vi "生成文本文件.vi"() -> ()   [LabVIEW 2013]
uses:
  <vilib>/Utility/file.llb/Write To Spreadsheet File (string).vi
panel:
  in  "字符串":string="1"
  in  "产品ID":string="201209190001"
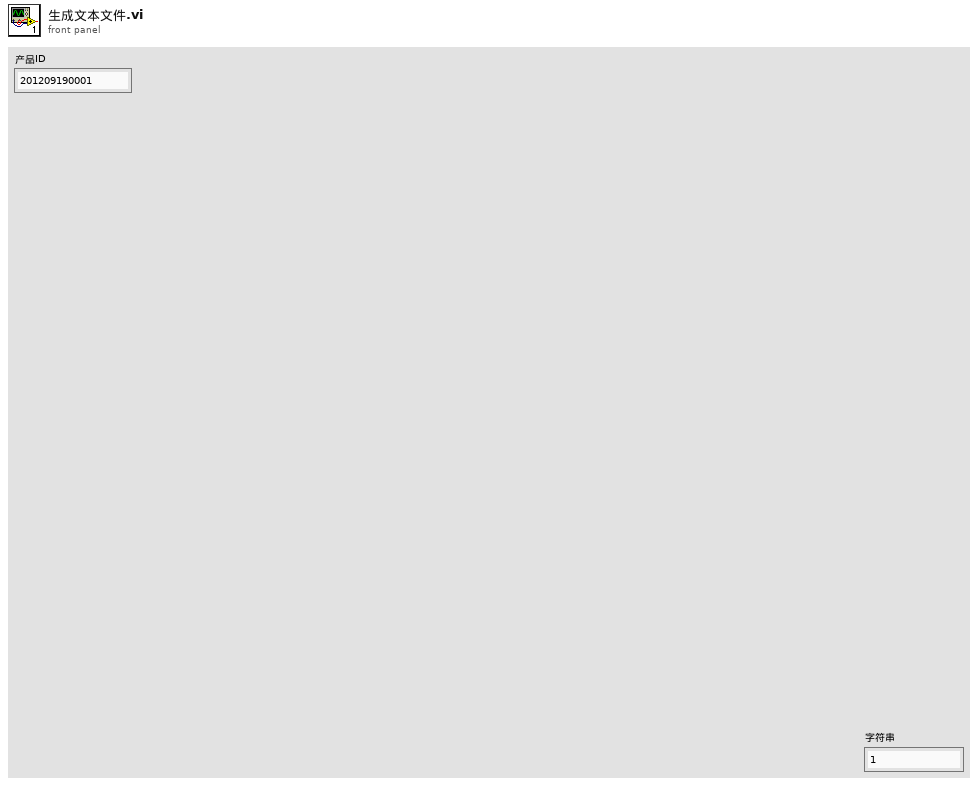
[diagram p1: front panel]
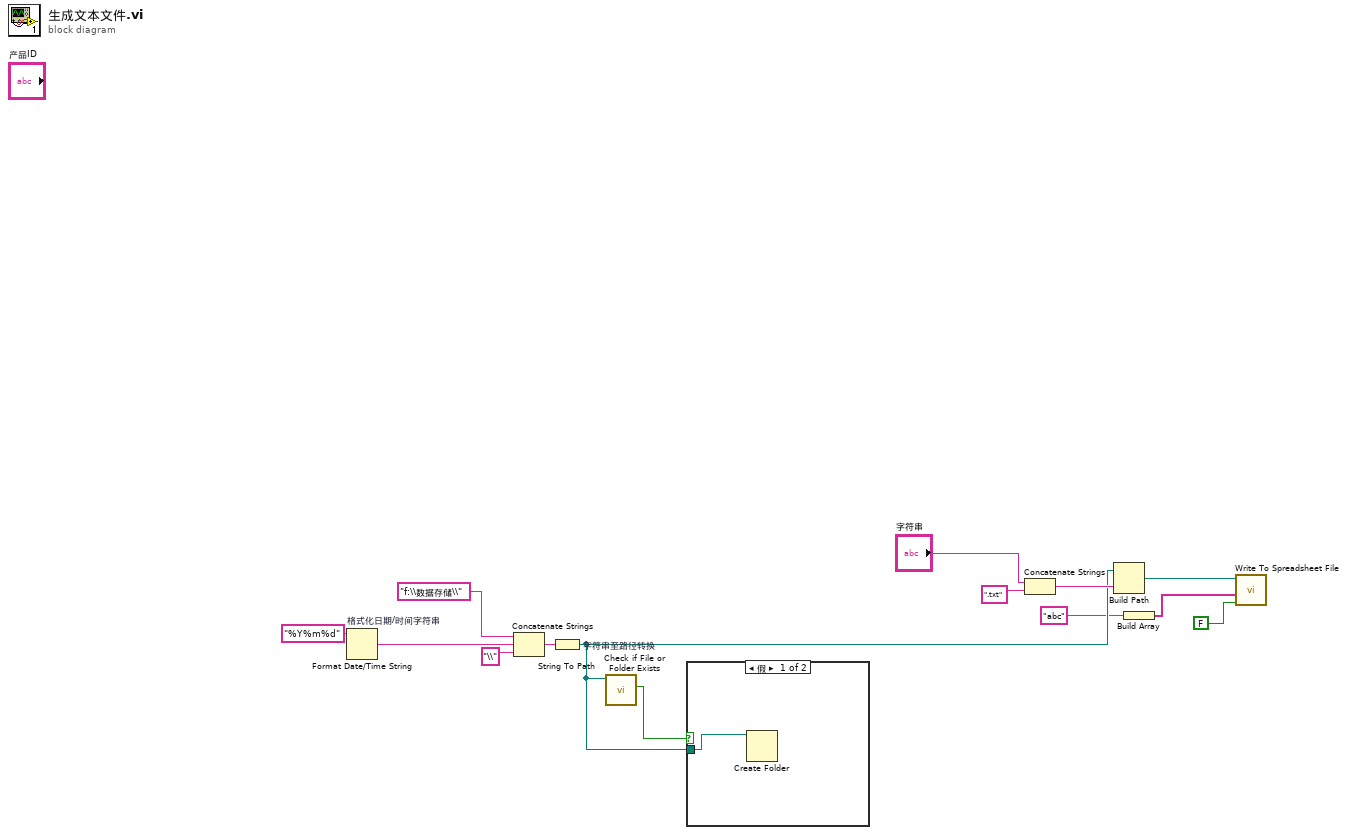
[diagram p0: block diagram]
diagram:
  n1 = Format Date/Time String "格式化日期/时间字符串"(time format string (%c)="%Y%m%d" ("时间格式字符串(%c)")) -> (date/time string=w5:string)  [unwired: 2 in]
  n2 = Concatenate Strings("f:\\数据存储\\" ("字符串"), w5, "\\" ("字符串")) -> (w11:string)
  n3 = String To Path "字符串至路径转换"(string=w11) -> (path=w4:path)
  n4 = call <vilib>:"Check if File or Folder Exists.vi"("path"=w4) -> ("file or folder exists?"=w6:bool)  [unwired: 8 in, 2 out]
  n5 = case shown="假" w6 {
    tunnel: w4 -> [w15 _]
    frame False {
      n6 = Create Folder(path (use dialog)=w15) -> ()  [unwired: 2 in, 3 out]
    }
    frame True {
    }
  }
  n7 = Concatenate Strings("字符串", ".txt" ("字符串")) -> (w8:string)
  n8 = Build Path(base path=w4, name or relative path=w8) -> (appended path=w7:path)
  n9 = Build Array("abc") -> (w2:string[])
  n10 = call-poly <vilib>:"Write To Spreadsheet File.vi"("append to file? (new file:F)"=FALSE, "1D data"=w2, "file path (dialog if empty)"=w7) -> ()  [unwired: 5 in, 1 out]
